vi "Rack.vi"(11 "Full System Configuration":T2 {"Ballast"."Side" max=5 step=1; "Ballast"."Small" max=5 step=1; "Ballast"."Main" max=5 step=1}) -> (3 "cluster":T1)   [LabVIEW 2023]
uses:
  Option Type Defs/Full System Configuration.ctl
  Option Type Defs/Rack.ctl
  Option Type Defs/Middle Rail.ctl
  Option Type Defs/Ballast.ctl
  Option Type Defs/Parts List.ctl
  <userlib>/_OpenG.lib/lvdata/lvdata.llb/openg_variant.lvlib
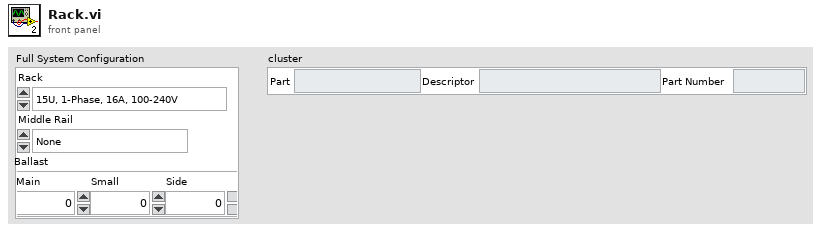
[diagram p1: front panel]
types:
  T1 = typedef "Parts List.ctl" = cluster{"Part":string, "Descriptor":string, "Part Number":string}
  T2 = typedef "Full System Configuration.ctl" = cluster{"Rack":T3, "Middle Rail":T4, "Ballast":T5}
  T3 = typedef "Rack.ctl" = enum16{"15U, 1-Phase, 16A, 100-240V", "15U, 1-Phase, 24A, 100-240V", "38U, 3-Phase Delta, 50A, 200-240V", "38U, 1-Phase, 24A, 100-120V", "38U, 3-Phase Wye, 50A, 200-240V", "38U, 3-Phase Delta, 50A, 380-480V", "38U, 3-Phase Delta, 32A, 200-240V", "38U, 3-Phase Wye, 16A, 100-240V", "44U, 1-Phase, 24A, 100-240V", "44U, 3-Phase Delta, 32A, 200-240V"}
  T4 = typedef "Middle Rail.ctl" = enum16{"None", "Flip Side Rear, D=168.83mm", "Parallel Rear, D=145mm", "Flip Side Front, D=145mm", "Parallel Front, D=145mm"}
  T5 = typedef "Ballast.ctl" = cluster{"Main":u16, "Small":u16, "Side":u16}
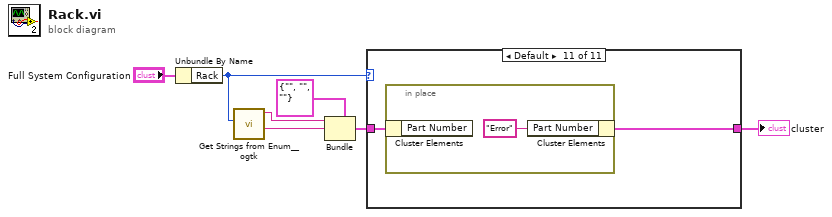
[diagram p0: block diagram]
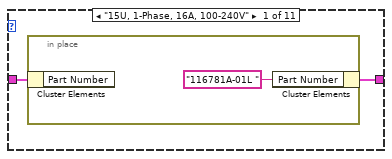
[diagram p2: hidden frame]
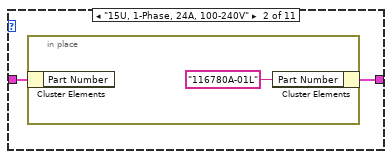
[diagram p3: hidden frame]
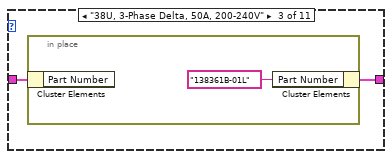
[diagram p4: hidden frame]
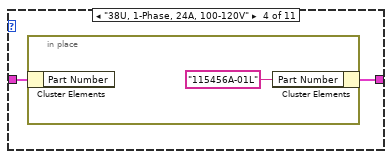
[diagram p5: hidden frame]
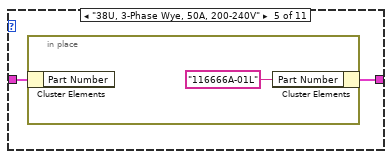
[diagram p6: hidden frame]
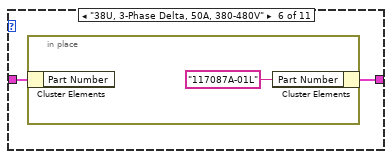
[diagram p7: hidden frame]
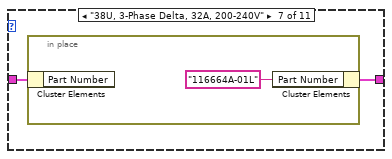
[diagram p8: hidden frame]
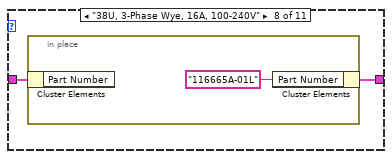
[diagram p9: hidden frame]
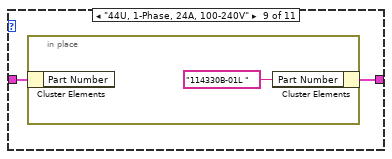
[diagram p10: hidden frame]
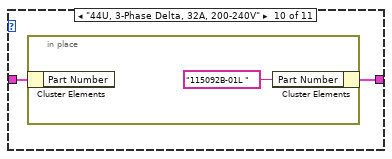
[diagram p11: hidden frame]
diagram:
  n1 = Unbundle By Name("Full System Configuration") -> ("Rack"=w7:T3)
  n2 = call <userlib>:"Get Strings from Enum__ogtk.vi"("Enum"=w7) -> ("String Value"=w1:string, "Enum Name"=w2:string)  [unwired: 7 in, 2 out]
  n3 = Bundle(cluster=T1 {"Part"="", "Descriptor"="", "Part Number"=""}, "Part"=w2, "Descriptor"=w1) -> (w4:T1)  [unwired: 1 in]
  n4 = case shown="Default" w7 {
    tunnel: w4 -> [w9 w12 w15 w18 w21 w24 w27 w30 w33 w36 w39]
    tunnel: [w8 w11 w14 w17 w20 w23 w26 w29 w32 w35 w38] -> w5
    frame "15U, 1-Phase, 16A, 100-240V" {
      n5 = in-place {
        n6 = in-place-cluster #1(w9) -> ()  [unwired: 1 out]
        n7 = in-place-cluster #1("Part Number"="116781A-01L ") -> (w8:T1)
      }
    }
    frame "15U, 1-Phase, 24A, 100-240V" {
      n8 = in-place {
        n9 = in-place-cluster #2(w12) -> ()  [unwired: 1 out]
        n10 = in-place-cluster #2("Part Number"="116780A-01L") -> (w11:T1)
      }
    }
    frame "38U, 3-Phase Delta, 50A, 200-240V" {
      n11 = in-place {
        n12 = in-place-cluster #3(w15) -> ()  [unwired: 1 out]
        n13 = in-place-cluster #3("Part Number"="138361B-01L") -> (w14:T1)
      }
    }
    frame "38U, 1-Phase, 24A, 100-120V" {
      n14 = in-place {
        n15 = in-place-cluster #4(w18) -> ()  [unwired: 1 out]
        n16 = in-place-cluster #4("Part Number"="115456A-01L") -> (w17:T1)
      }
    }
    frame "38U, 3-Phase Wye, 50A, 200-240V" {
      n17 = in-place {
        n18 = in-place-cluster #5(w21) -> ()  [unwired: 1 out]
        n19 = in-place-cluster #5("Part Number"="116666A-01L") -> (w20:T1)
      }
    }
    frame "38U, 3-Phase Delta, 50A, 380-480V" {
      n20 = in-place {
        n21 = in-place-cluster #6(w24) -> ()  [unwired: 1 out]
        n22 = in-place-cluster #6("Part Number"="117087A-01L") -> (w23:T1)
      }
    }
    frame "38U, 3-Phase Delta, 32A, 200-240V" {
      n23 = in-place {
        n24 = in-place-cluster #7(w27) -> ()  [unwired: 1 out]
        n25 = in-place-cluster #7("Part Number"="116664A-01L") -> (w26:T1)
      }
    }
    frame "38U, 3-Phase Wye, 16A, 100-240V" {
      n26 = in-place {
        n27 = in-place-cluster #8(w30) -> ()  [unwired: 1 out]
        n28 = in-place-cluster #8("Part Number"="116665A-01L") -> (w29:T1)
      }
    }
    frame "44U, 1-Phase, 24A, 100-240V" {
      n29 = in-place {
        n30 = in-place-cluster #9(w33) -> ()  [unwired: 1 out]
        n31 = in-place-cluster #9("Part Number"="114330B-01L ") -> (w32:T1)
      }
    }
    frame "44U, 3-Phase Delta, 32A, 200-240V" {
      n32 = in-place {
        n33 = in-place-cluster #10(w36) -> ()  [unwired: 1 out]
        n34 = in-place-cluster #10("Part Number"="115092B-01L ") -> (w35:T1)
      }
    }
    frame Default {
      n35 = in-place {
        n36 = in-place-cluster #11(w39) -> ()  [unwired: 1 out]
        n37 = in-place-cluster #11("Part Number"="Error") -> (w38:T1)
      }
    }
  }
  "cluster" <- w5
